vi "Scenarios.vi"() -> ()   [LabVIEW 2015]
uses:
  <vilib>/httpClient/LabVIEWHTTPClient.lvlib
panel:
  in  "String 5":string
  in  "String 4":string
  in  "String 3":string
  in  "String 2":string
  in  "OK Button 4":bool
  in  "OK Button 2":bool
  in  "String":string
  # "Entrer Nom du Scénario"
  # "Entrer Date de début du Scénario"
  # "Entrer Date de fin du Scénario"
  # "Entrer Heure de début du Scénario"
  # "Entrer Heure de fin du Scénario"
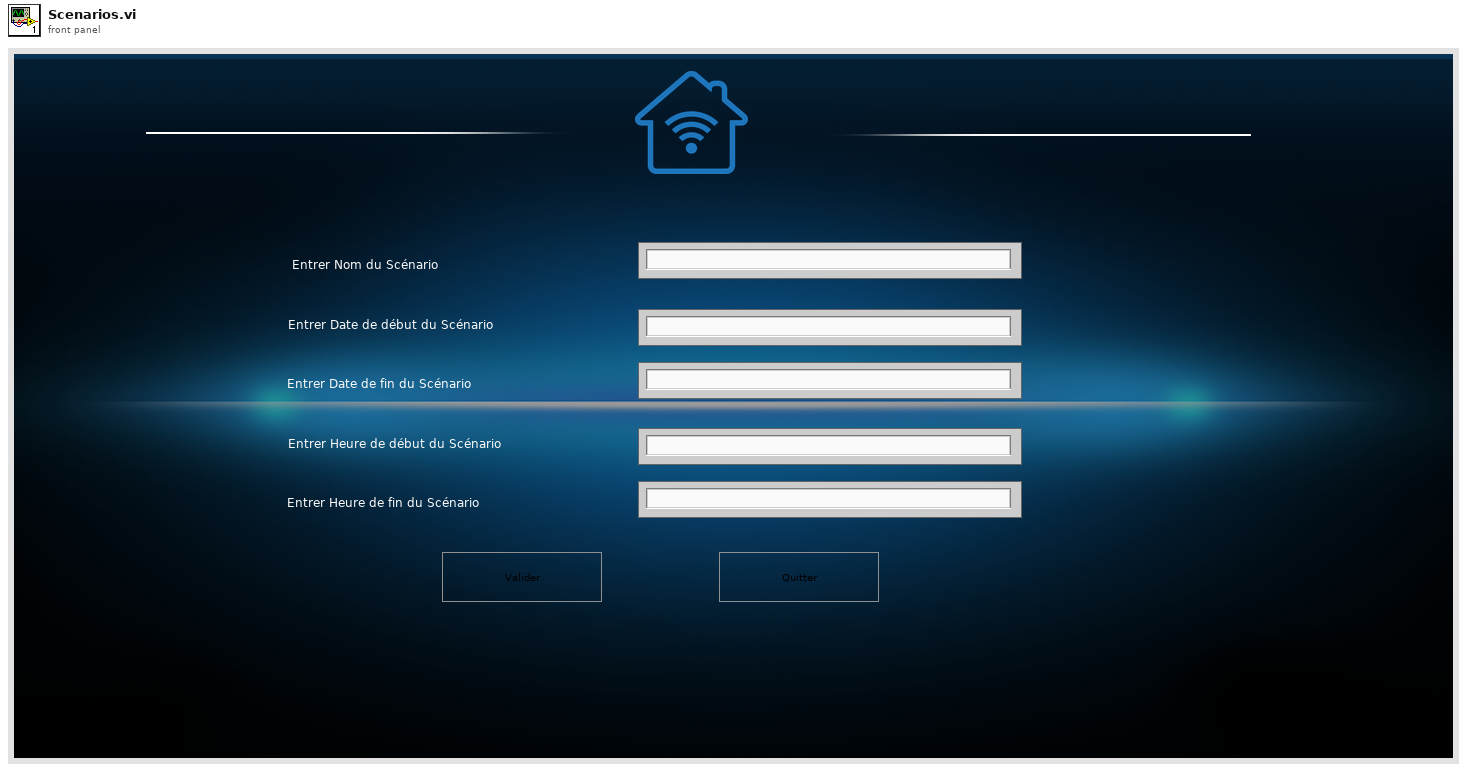
[diagram p1: front panel]
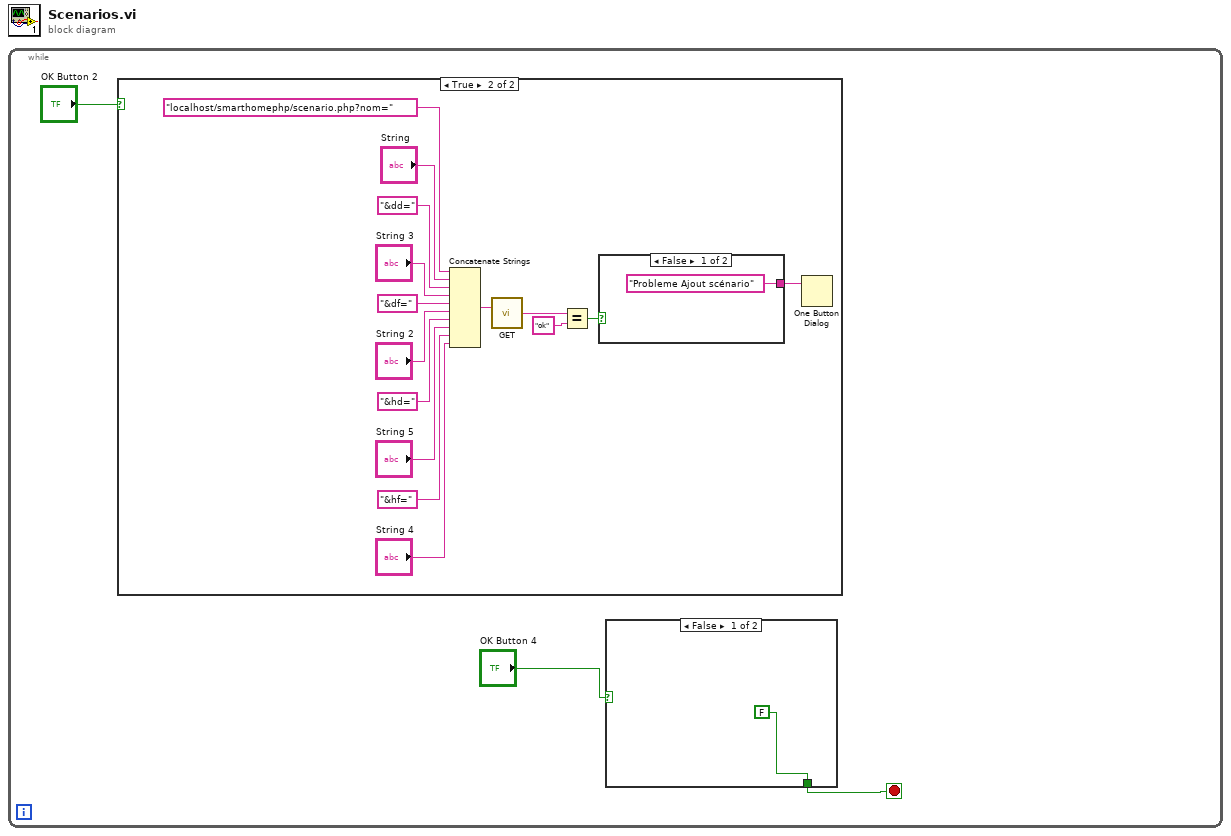
[diagram p0: block diagram]
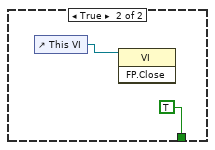
[diagram p2: hidden frame]
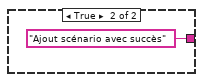
[diagram p4: hidden frame]
diagram:
  n1 = while {
    stop <- w2 stop-if-true
    n2 = case shown="True" "OK Button 2" {
      frame False {
      }
      frame True {
        n3 = Concatenate Strings("localhost/smarthomephp/scenario.php?nom=", "String", "&dd=", "String 3", "&df=", "String 2", "&hd=", "String 5", "&hf=", "String 4") -> (w11:string)
        n4 = call <vilib>:"GET.vi"("url"=w11) -> ("body"=w10:string)  [unwired: 11 in, 3 out]
        n5 = Equal?(x=w10, y="ok") -> (x = y?=w8:bool)
        n6 = case shown="False" w8 {
          tunnel: ["Probleme Ajout scénario" "Ajout scénario avec succès"] -> w7
          frame False {
          }
          frame True {
          }
        }
        n7 = One Button Dialog(message=w7) -> ()  [unwired: 1 in, 1 out]
      }
    }
    n8 = case shown="False" "OK Button 4" {
      tunnel: [FALSE TRUE] -> w2
      frame False {
      }
      frame True {
        n9 = control-ref of="This VI"() -> (w6:refnum<vi>)
        n10 = invoke class="VI" method="FP.Close"(reference=w6) -> ()  [unwired: 2 in, 3 out]
      }
    }
  }
